vi "Begin.vi"() -> (0 "Error Out":errorcluster)   [LabVIEW 2020]
doc: "This VI opens device references, sets constants, clears hardware sticky faults, defines static VI references, and resets gobal variables."
uses:
  <vilib>/Rock Robotics/WPI/DriverStation/WPI_DriverStationRobotMode2.ctl
  GlobalDriverStationData.vi
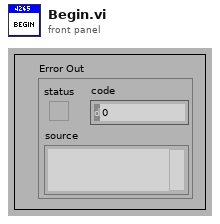
[diagram p1: front panel]
types:
  T1 = typedef "WPI_DriverStationRobotMode2.ctl" = enum16{"Autonomous Disabled", "Autonomous Enabled", "Teleop Disabled", "Teleop Enabled", "Disconnected", "Finish", "Test Disabled", "Test Enabled", "Emergency Stopped"}
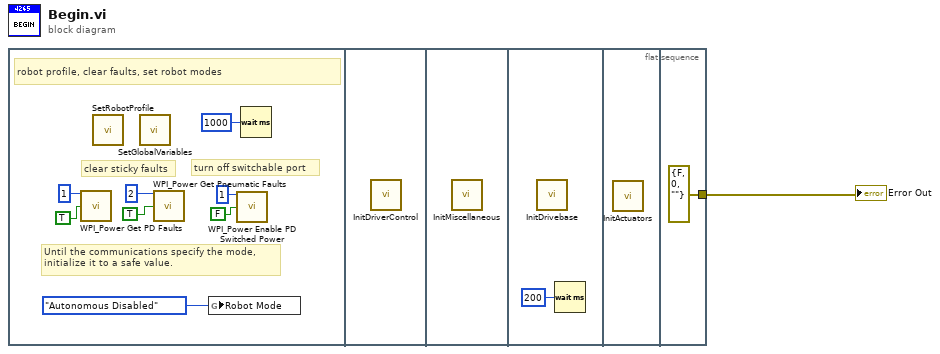
[diagram p0: block diagram]
diagram:
  n1 = flat-sequence {
    tunnel: [errorcluster {"status"=FALSE, "code"=0, "source"=""} ("error in")] -> w1
    frame #0 {
      # "turn off switchable port"
      # "clear sticky faults"
      # "Until the communications specify the mode,\ninitialize it to a safe value."
      # "robot profile, clear faults, set robot modes"
      n2 = call <vilib>:"WPI_Power Get PD Faults.vi"("Power Distribution (def)"=u8 1 ("Power Distribution Panel (0)"), "Clear Sticky Faults"=TRUE) -> ()  [unwired: 10 in, 4 out]
      n3 = call "SetRobotProfile.vi"() -> ()  [unwired: 1 in]
      n4 = call "SetGlobalVariables.vi"() -> ()  [unwired: 1 in]
      n5 = call <vilib>:"WPI_Power Get Pneumatic Faults.vi"("Pneumatics device (def)"=u8 2 ("Pneumatics Control Module (0)"), "Clear Sticky Faults"=TRUE) -> ()  [unwired: 8 in, 6 out]
      n6 = global write "GlobalDriverStationData.vi" "Robot Mode"(WPI_DriverStationRobotMode2."Autonomous Disabled" ("Robot Mode")) -> ()
      n7 = call <vilib>:"WPI_Power Enable PD Switched Power.vi"("Power Distribution (def)"=u8 1, "Switch Channel Value"=FALSE) -> ()  [unwired: 12 in, 2 out]
      n8 = Wait (ms)(milliseconds to wait=u32 1000) -> ()  [unwired: 1 out]
    }
    frame #1 {
      n9 = call "InitDriverControl.vi"() -> ()  [unwired: 1 in]
    }
    frame #2 {
      n10 = call "InitMiscellaneous.vi"() -> ()  [unwired: 1 in]
    }
    frame #3 {
      n11 = call "InitDrivebase.vi"() -> ()  [unwired: 1 in]
      n12 = Wait (ms)(milliseconds to wait=u32 200) -> ()  [unwired: 1 out]
    }
    frame #4 {
      n13 = call "InitActuators.vi"() -> ()  [unwired: 1 in]
    }
    frame #5 {
    }
  }
  "Error Out" <- w1
